vi "disable.vi"(8 "error in (no error)":errorcluster, 11 "GenericEmissionSensor in":refnum<class "DetectorYK090623DAQmxAnalog.lvclass">) -> (0 "error out":errorcluster, 3 "GenericEmissionSensor out":refnum<class "DetectorYK090623DAQmxAnalog.lvclass">)   [LabVIEW 2010, in "DetectorYK090623DAQmxAnalog.lvclass"]
uses:
  DetectorYK090623DAQmxAnalog.lvclass
  DetectorYK090623DAQmxAnalog.lvclass/DetectorYK090623DAQmxAnalog.ctl
  AnalogOut/AnalogOutDL101207DAQmx/AnalogOutDL101207DAQmx/AnalogOutDL101207DAQmx.lvclass
  GenericDetector/GenericDetector/GenericDetector.lvclass
  common/classes/ErrorController/ErrorController/class_data.vi
  common/classes/ErrorController/ErrorController/ErrorController.lvclass
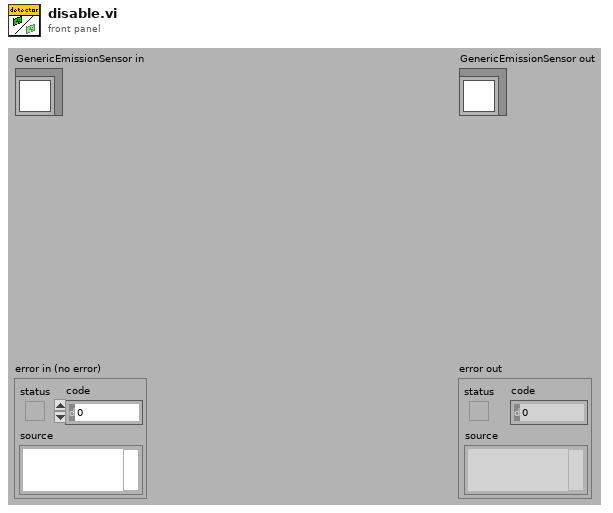
[diagram p1: front panel]
types:
  T1 = typedef "GenericDetector.lvclass/status_enum.ctl" = enum16{"disabled", "enabled"}
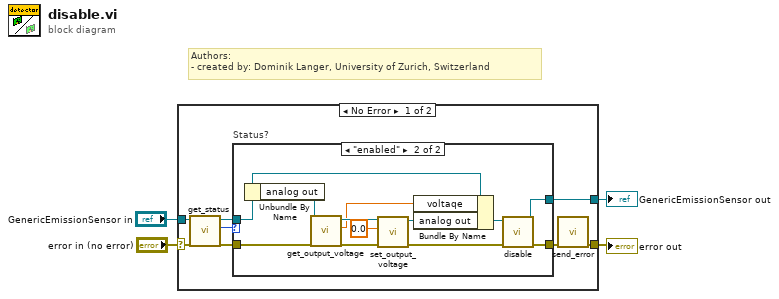
[diagram p0: block diagram]
diagram:
  # "Authors: \n- created by: Dominik Langer, University of Zurich, Switzerland"
  n1 = case shown="No Error" "error in (no error)" {
    selector: "error in (no error)" -> [w11 w28]
    tunnel: "GenericEmissionSensor in" -> [w9 w27]
    tunnel: [w6 w28] -> w2
    tunnel: [w12 w27] -> w1
    frame No Error {
      n2 = call-dynamic "get_status.vi"("error in (no error)"=w11, "GenericEmissionSensor.lvclass in"=w9) -> ("error out"=w10:errorcluster, "status"=w7:T1, "GenericEmissionSensor.lvclass out"=w8:refnum<class "DetectorYK090623DAQmxAnalog.lvclass">)  [unwired: 7 out]
      n3 = case "Status?" shown="\"enabled\"" w7 {
        tunnel: [w13 w22] -> w5
        tunnel: [w14 w21] -> w12
        tunnel: w10 -> [w13 w16]
        tunnel: w8 -> [w14 w15]
        frame "disabled", Default {
          # "Nothing to be done if it's already disabled..."
        }
        frame "enabled" {
          n4 = Unbundle By Name(w15) -> ("analog out"=w19:refnum<class "AnalogOutDL101207DAQmx.lvclass">)
          n5 = call-dynamic "get_output_voltage.vi"("error in (no error)"=w16, "DAQmxAnalogOut.lvclass in"=w19) -> ("error out"=w20:errorcluster, "current voltage"=w17:dbl[unit], "DAQmxAnalogOut.lvclass out"=w18:refnum<class "AnalogOutDL101207DAQmx.lvclass">)  [unwired: 7 in]
          n6 = call-dynamic "set_output_voltage.vi"("error in (no error)"=w20, "output value"=dbl[unit] 0.0, "DAQmxAnalogOut in"=w18) -> ("error out"=w25:errorcluster, "DAQmxAnalogOut out"=w24:refnum<class "AnalogOutDL101207DAQmx.lvclass">)  [unwired: 7 in]
          n7 = Bundle By Name(cluster=w15, "voltaqe"=w17, "analog out"=w24) -> (w23:refnum<class "DetectorYK090623DAQmxAnalog.lvclass">)
          n8 = call-parent "disable.vi"("error in (no error)"=w25, "GenericEmissionSensor in"=w23) -> ("error out"=w22:errorcluster, "GenericEmissionSensor out"=w21:refnum<class "DetectorYK090623DAQmxAnalog.lvclass">)  [unwired: 8 out]
        }
      }
      n9 = call "send_error.vi"("error in (no error)"=w5) -> ("error out"=w6:errorcluster)  [unwired: 10 in]
    }
    frame Error {
    }
  }
  "error out" <- w2
  "GenericEmissionSensor out" <- w1
